vi "ConvertTextBasedCodeToLabVIEW_FixExpressionBodied.vi"(11 "Expression-bodiedTextIn":string="public virtual void Send(string message) => this.mediator.Send(message, this);\n\npublic void DisplayName() => Console.WriteLine(ToString());\n\npublic virtual void Send(string message) => this.mediator.Send(message, this);") -> (3 "ModifiedExpression-bodiedTextOut":string)   [LabVIEW 2020]
uses:
  <vilib>/regexp/Match Regular Expression.xnode
panel:
  # "public override string ToString() => $\"{fname} {lname}\".Trim();\n public override string ToString() {=> $\"{fname} {lname}\".Trim();}\n\npublic void DisplayName() => Console.WriteLine(ToString());\npublic void DisplayName() { => Console.WriteLine(ToString());}\n\npublic virtual void Send(string message) => this.mediator.Send(message, this);\npublic virtual void Send(string message) {=> this.mediator.Send(message, this);}"
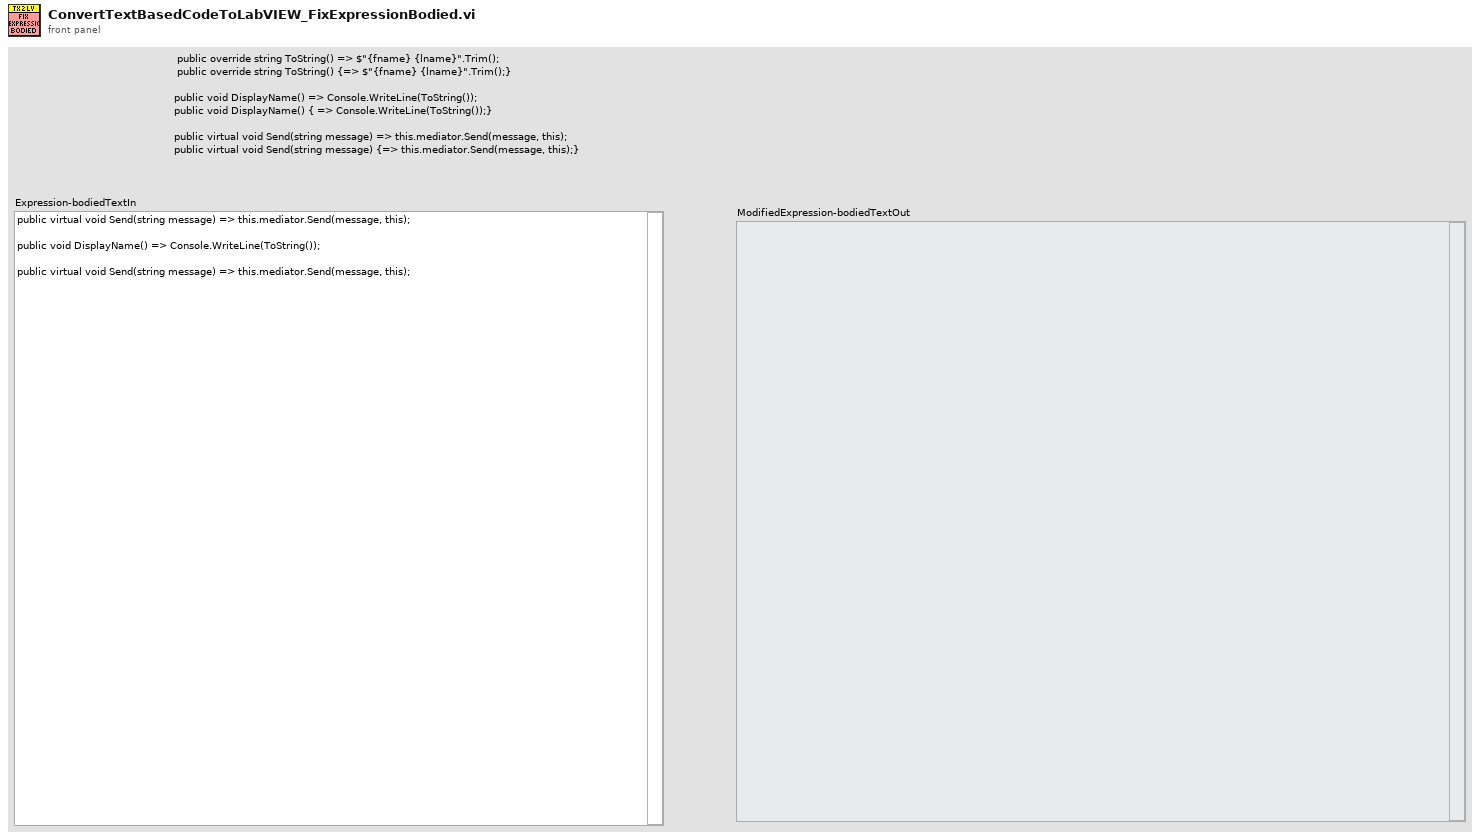
[diagram p1: front panel]
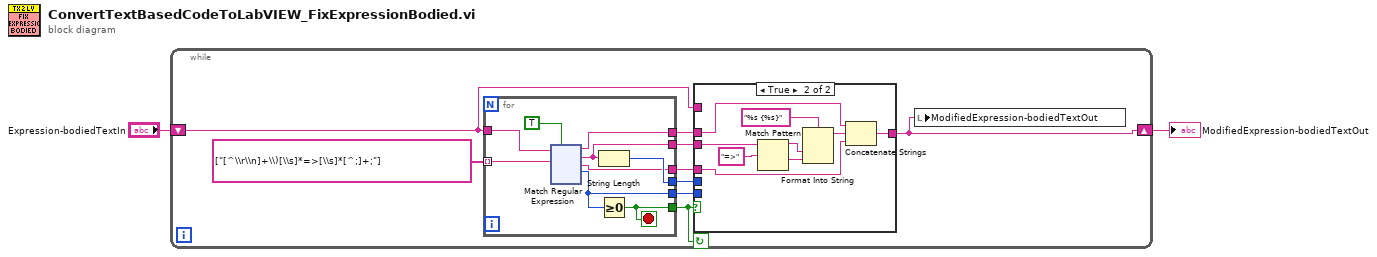
[diagram p0: block diagram]
diagram:
  n1 = while {
    shift-right: [w6] -> w1
    shift-left: "Expression-bodiedTextIn" -> [w9]
    stop <- w8 continue-if-true
    n2 = for {
      tunnel: string[] ["[^\\r\\n]+\\)[\\s]*=>[\\s]*[^;]+;"] ("input string") -> [w29] mode=indexing
      tunnel: w9 -> [w28]
      tunnel: [w27] -> w10
      tunnel: [w26] -> w8
      tunnel: [w25] -> w7
      tunnel: [w24] -> w5
      tunnel: [w22] -> w4
      tunnel: [w23] -> w3
      stop <- w26 stop-if-true
      n3 = xnode "Match Regular Expression"("input string"=w28, "regular expression"=w29, "ignore case? (F)"=TRUE) -> ("before match"=w23:string, "whole match"=w24:string, "after match"=w22:string, "offset past match"=w27:i32)  [unwired: 3 in, 1 out]
      n4 = String Length(string=w24) -> (length=w25:i32)
      n5 = Greater Or Equal To 0?(x=w27) -> (x >= 0?=w26:bool)
    }
    n6 = case shown="True" w8 {
      tunnel: w10 -> [_ _]
      tunnel: w9 -> [w12 _]
      tunnel: [w12 w21] -> w6
      tunnel: w7 -> [_ _]
      tunnel: w5 -> [_ w14]
      tunnel: w4 -> [_ w19]
      tunnel: w3 -> [_ w20]
      frame False {
      }
      frame True {
        n7 = Match Pattern(string=w14, regular expression="=>") -> (before substring=w17:string, after substring=w15:string)  [unwired: 1 in, 2 out]
        n8 = Format Into String(format string="%s {%s}", w17, w15) -> (resulting string=w13:string)  [unwired: 2 in, 1 out]
        n9 = Concatenate Strings(w20, w13, w19) -> (w21:string)
      }
    }
    n10 = local write "ModifiedExpression-bodiedTextOut"(w6) -> ()
  }
  "ModifiedExpression-bodiedTextOut" <- w1
